vi "LightLoop.vi"   [LabVIEW 2018]
uses:
  <vilib>/Platform/TimedLoop/XDataNode/timing_clust.ctl
  <vilib>/Platform/TimedLoop/XDataNode/nitl_modes.ctl
  <vilib>/Platform/TimedLoop/XDataNode/wakeup.ctl
  <vilib>/platform/TimedLoop/XDataNode/XDataNode.xnode
  <vilib>/Platform/TimedLoop/XDataNode/XDNodeRunTimeDep.lvlib
types:
  T1 = typedef "WPI_MotorControlDeviceRef.ctl" = cluster{"DeviceStatus":errorcluster, "Type":T2, "PWM":cluster{"PWM Channel":T3, "DeadBand":T4}, "CAN":cluster{"Device Number":u8, "SetOutput VI Ref":variant, "GetOutput VI Ref":variant, "Enable VI Ref":variant, "Disable VI Ref":variant, "Data":variant}, "Invert":bool, "DIO PWM":cluster{"PWM \"Enable\" Channel":T3, "DIOChannel":T5, "PWM Rate":dbl}}
  T2 = typedef "WPI_MotorControlType.ctl" = enum16{"PWM", "CAN", "DIO PWM"}
  T3 = typedef "FPGA_DIOPWMChannel.ctl" = enum8{"PWM 0", "PWM 1", "PWM 2", "PWM 3", "PWM 4", "PWM 5", "PWM 6", "PWM 7", "PWM 8", "PWM 9", "PWM MXP 0", "PWM MXP 1", "PWM MXP 2", "PWM MXP 3", "PWM MXP 4", "PWM MXP 5", "PWM MXP 6", "PWM MXP 7", "PWM MXP 8", "PWM MXP 9", "Invalid"}
  T4 = typedef "WPI_PWMDeadband.ctl" = cluster{"Name":string, "maxPositivePwm":i32, "minPositivePwm":i32, "centerPwm":i32, "maxNegativePwm":i32, "minNegativePwm":i32, "angularRange":u16}
  T5 = typedef "FPGA_DIOChannel.ctl" = enum8{"DIO 0", "DIO 1", "DIO 2", "DIO 3", "DIO 4", "DIO 5", "DIO 6", "DIO 7", "DIO 8", "DIO 9", "DIO MXP 0", "DIO MXP 1", "DIO MXP 2", "DIO MXP 3", "DIO MXP 4", "DIO MXP 5", "DIO MXP 6", "DIO MXP 7", "DIO MXP 8", "DIO MXP 9", "DIO MXP 10", "DIO MXP 11", "DIO MXP 12", "DIO MXP 13", "DIO MXP 14", "DIO MXP 15", "SPI Port CS1", "SPI Port CS2", "SPI Port CS3", "SPI Port MISO", "SPI Port MOSI", "Invalid"}
  T6 = typedef "XDNodeRunTimeDep.lvlib/timing_clust.ctl" = cluster{"Expected End [f-1]":u64, "Actual End [f-1]":u64, "Finished Late? [f-1]":bool, "Expected End [i-1]":u64, "Actual End [i-1]":u64, "Finished Late? [i-1]":bool, "Expected Start [i]":u64, "Actual Start [i]":u64, "Expected Start [f]":u64, "Actual Start [f]":u64, "Source Name":string, "Structure Name":string, "Period":i64, "Deadline":i64, "Offset":i64, "Start":i64, "Priority":i32, "Timeout":i32, "Mode":T7, "Wakeup Reason":T8, "Error":errorcluster, "Source Type":string, "Secondary Source Type":string, "Global End Time":u64, "Global Start Time":u64, "Frame Duration":u64, "Iteration Duration":u64, "Assigned CPU":i32, "I/O Scan Engine Mode":u32}
  T7 = typedef "XDNodeRunTimeDep.lvlib/nitl_modes.ctl" = enum32{"No Change", "Process missed periods, maintain original phase", "Discard missed periods, maintain original phase", "Process missed periods, ignore original phase", "Discard missed periods, ignore original phase"}
  T8 = typedef "XDNodeRunTimeDep.lvlib/wakeup.ctl" = enum32{"Normal", "Aborted", "Asynchronous wakeup", "Timing source error", "Timed loop error", "Timeout"}
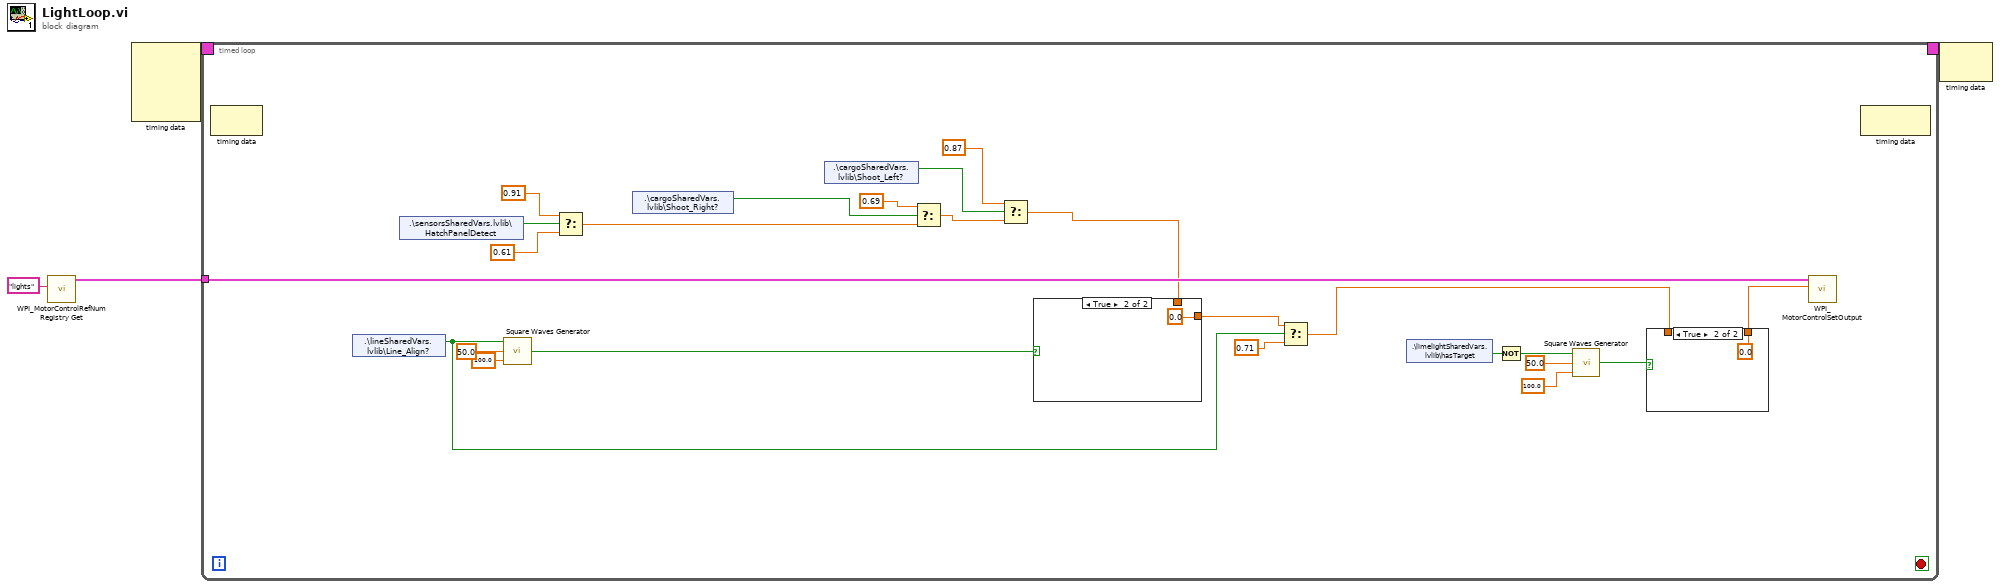
[diagram p0: block diagram]
diagram:
  n1 = call <vilib>:"WPI_MotorControlRefNum Registry Get.vi"("refnum name"="lights") -> ("MotorControlDevRef"=w1:T1)  [unwired: 9 in, 1 out]
  n2 = node-c288() -> (w4:T6)  [unwired: 4 in]
  n3 = timed-loop {
    timing: w4 -> [_]
    timing-out: [_] -> w3
    tunnel: w1 -> [w20]
    stop <- _ stop-if-true
    n4 = node-c288() -> ()  [unwired: 1 in, 1 out]
    n5 = shared-variable ".\\lineSharedVars.lvlib\\Line_Align?"() -> (w22:bool)  [unwired: 1 in, 1 out]
    n6 = shared-variable ".\\sensorsSharedVars.lvlib\\HatchPanelDetect"() -> (w28:bool)  [unwired: 1 in, 1 out]
    n7 = call <userlib>:"Square Waves Generator.vi"("Duty Cycle (%)"=100.0, "Period (ms)"=50.0, "Enable"=w22) -> ("Signal"=w24:bool)
    n8 = Select(t=0.91, s=w28, f=0.61) -> (s? t:f=w8:dbl)
    n9 = shared-variable ".\\cargoSharedVars.lvlib\\Shoot_Right?"() -> (w7:bool)  [unwired: 1 in, 1 out]
    n10 = shared-variable ".\\cargoSharedVars.lvlib\\Shoot_Left?"() -> (w10:bool)  [unwired: 1 in, 1 out]
    n11 = Select(t=0.69, s=w7, f=w8) -> (s? t:f=w9:dbl)
    n12 = Select(t=0.87, s=w10, f=w9) -> (s? t:f=w11:dbl)
    n13 = case shown="True" w24 {
      tunnel: [w31 0.0] -> w23
      tunnel: w11 -> [w31 _]
      frame False {
      }
      frame True {
      }
    }
    n14 = Select(t=w23, s=w22, f=0.71 ("Output")) -> (s? t:f=w15:dbl)
    n15 = shared-variable ".\\limelightSharedVars.lvlib\\hasTarget"() -> (w17:bool)  [unwired: 1 in, 1 out]
    n16 = Not(x=w17) -> (.not. x?=w16:bool)
    n17 = call <userlib>:"Square Waves Generator.vi"("Duty Cycle (%)"=100.0, "Period (ms)"=50.0, "Enable"=w16) -> ("Signal"=w18:bool)
    n18 = case shown="True" w18 {
      tunnel: [w29 0.0 ("Output")] -> w14
      tunnel: w15 -> [w29 _]
      frame False {
      }
      frame True {
      }
    }
    n19 = call <vilib>:"WPI_MotorControlSetOutput.vi"("Output"=w14, "MotorControlDevRef"=w20) -> ()  [unwired: 7 in, 3 out]
    n20 = node-c288() -> ()  [unwired: 1 in, 1 out]
  }
  n21 = node-c288(w3) -> ()  [unwired: 1 out]
